vi "Remove_spikes_Single_ch.vi"(0 "LDA data":dbl[][](array[numeric]) format="%.3f", 1 "Sigma cut":i32, 2 "BSA Channels":T1(array[ring]), 3 "LDA numder":enum16{"LDA 1", "LDA 2"}(ring)) -> (5 "Filtered data":dbl[][](array[numeric]) format="%.3f", 6 "No of points removed":i32)   [LabVIEW 2010]
uses:
  Globals/LDA_meas_global_1.vi
  Globals/LDA_meas_global_2.vi
  <vilib>/Analysis/NI_AALBase.lvlib
panel:
  out "No of points outside range":i32
  out "Sigma":dbl[](array[numeric]) format="%.4f"
  out "Points removed":i32[](array[numeric])
  out "output":dbl[][](graph)
  out "input":dbl[][](graph)
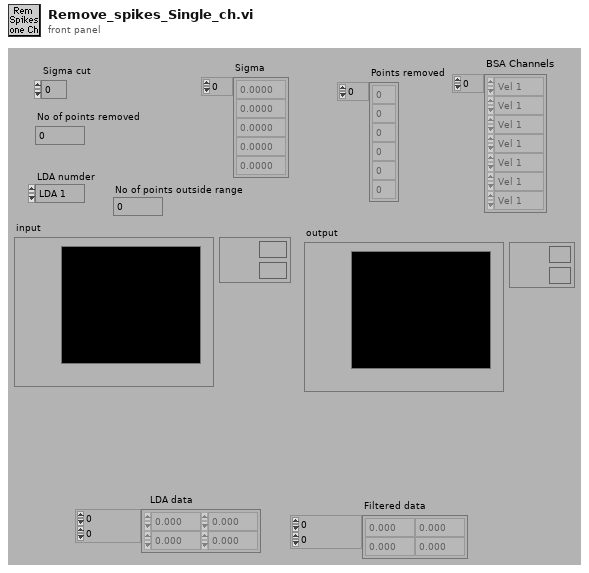
[diagram p1: front panel]
types:
  T1 = enum16{"Vel 1", "Trans 1", "Arr 1", "Vel 2", "Trans 2", "Arr 2", "Index"}[]
  T2 = enum16{"Vel 1", "Trans 1", "Arr 1", "Vel 2", "Trans 2", "Arr 2", "Index"}
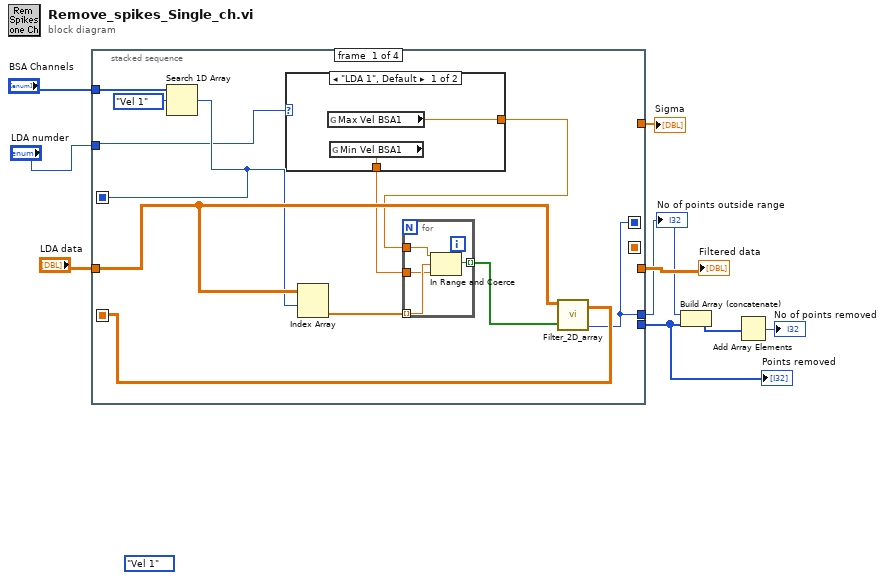
[diagram p0: block diagram]
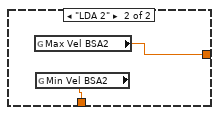
[diagram p2: hidden frame]
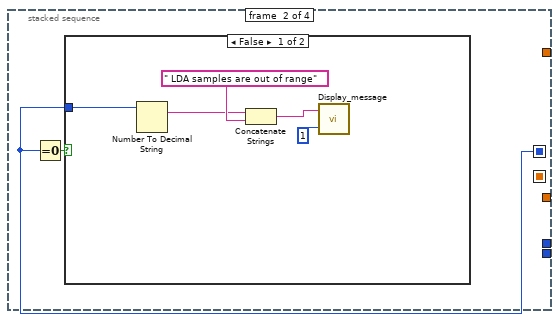
[diagram p3: hidden frame]
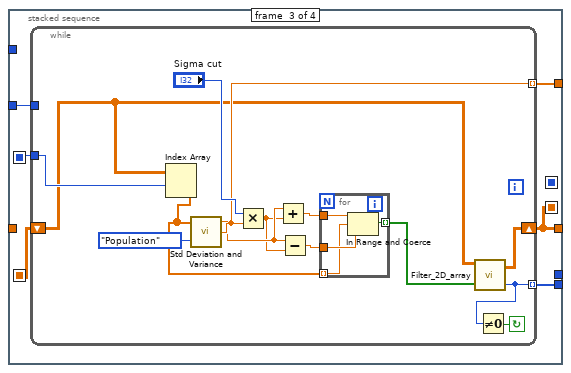
[diagram p5: hidden frame]
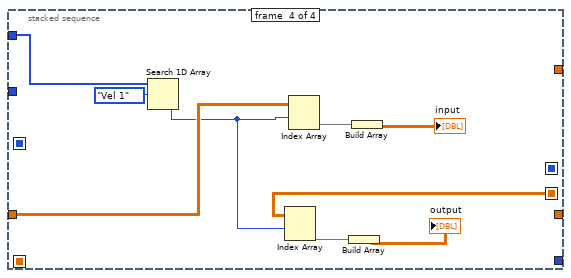
[diagram p6: hidden frame]
diagram:
  (unwired) T2."Vel 1"
  n1 = stacked-sequence {
    seq-local: [w19 _ _ _] -> [_ _ w38 _]
    seq-local: [w18 _ _ _] -> [_ w29 _ _]
    seq-local: [w14 _ _ _] -> [_ _ w37 _]
    seq-local: [_ _ w36 _] -> [_ _ _ w66]
    tunnel: [_ _ w41 _] -> w6
    tunnel: [_ _ w36 _] -> w7
    tunnel: "LDA data" -> [w20 _ _ w67]
    tunnel: [_ _ w40 _] -> w3
    tunnel: "LDA numder" -> [w13 _ w39 _]
    tunnel: [w18 _ _ _] -> w5
    tunnel: "BSA Channels" -> [w17 _ _ w68]
    frame #0 {
      n2 = Search 1D Array(1D array=w17, element=T2."Vel 1") -> (index of element=w14:i32)  [unwired: 1 out]
      n3 = case shown="\"LDA 1\", Default" w13 {
        tunnel: [w22 w24] -> w11
        tunnel: [w21 w23] -> w10
        frame "LDA 1", Default {
          n4 = global read "LDA_meas_global_1.vi" "Max Vel BSA1"() -> (w22:dbl)
          n5 = global read "LDA_meas_global_1.vi" "Min Vel BSA1"() -> (w21:dbl)
        }
        frame "LDA 2" {
          n6 = global read "LDA_meas_global_2.vi" "Max Vel BSA2"() -> (w24:dbl)
          n7 = global read "LDA_meas_global_2.vi" "Min Vel BSA2"() -> (w23:dbl)
        }
      }
      n8 = Index Array(array=w20, index (row)=w14) -> (element=w16:dbl[])  [unwired: 1 in]
      n9 = for {
        tunnel: w16 -> [w28] mode=indexing
        tunnel: [w27] -> w12 mode=indexing
        tunnel: w11 -> [w26]
        tunnel: w10 -> [w25]
        n10 = In Range and Coerce(upper limit=w26, x=w28, lower limit=w25) -> (In Range?=w27:bool)  [unwired: 1 out]
      }
      n11 = call "Filter_2D_array.vi"("All 2D data"=w20, "Accept array"=w12) -> ("Filtered data"=w19:dbl[][], "No of points removed"=w18:i32)  [unwired: 3 out]
    }
    frame #1 {
      n12 = Equal To 0?(x=w29) -> (x = 0?=w30:bool)
      n13 = case shown="False" w30 {
        tunnel: w29 -> [w35 _]
        frame False {
          n14 = Number To Decimal String(number=w35) -> (decimal integer string=w31:string)  [unwired: 1 out]
          n15 = Concatenate Strings(w31, " LDA samples are out of range") -> (w34:string)
          n16 = call "Display_message.vi"("Time to display message"=1, "Message"=w34) -> ()  [unwired: 2 out]
        }
        frame True {
        }
      }
    }
    frame #2 {
      n17 = while {
        tunnel: w37 -> [w50]
        tunnel: [w51] -> w41 mode=indexing
        tunnel: [w53] -> w40 mode=indexing
        tunnel: w39 -> [_]
        shift-left: w38 -> [w49]
        shift-right: [w55] -> w36
        stop <- w54 continue-if-true
        n18 = Index Array(array=w49, index (row)=w50) -> (element=w44:dbl[])  [unwired: 1 in]
        n19 = call <vilib>:"Std Deviation and Variance.vi"("X"=w44, "Weighting (Sample)"=enum16{"Sample", "Population"}."Population") -> ("mean"=w48:dbl, "standard deviation"=w51:dbl)  [unwired: 1 out]
        n20 = Multiply(x="Sigma cut", y=w51) -> (x*y=w45:dbl)
        n21 = Add(x=w48, y=w45) -> (x+y=w46:dbl)
        n22 = Subtract(x=w48, y=w45) -> (x-y=w47:dbl)
        n23 = for {
          tunnel: w46 -> [w59]
          tunnel: w47 -> [w58]
          tunnel: w44 -> [w57] mode=indexing
          tunnel: [w56] -> w43 mode=indexing
          n24 = In Range and Coerce(upper limit=w59, x=w57, lower limit=w58) -> (In Range?=w56:bool)  [unwired: 1 out]
        }
        n25 = call "Filter_2D_array.vi"("All 2D data"=w49, "Accept array"=w43) -> ("Filtered data"=w55:dbl[][], "No of points removed"=w53:i32)  [unwired: 3 out]
        n26 = Not Equal To 0?(x=w53) -> (x != 0?=w54:bool)
      }
    }
    frame #3 {
      n27 = Search 1D Array(1D array=w68, element=T2."Vel 1") -> (index of element=w62:i32)  [unwired: 1 out]
      n28 = Index Array(array=w66, index (row)=w62) -> (element=w60:dbl[])  [unwired: 1 in]
      n29 = Index Array(array=w67, index (row)=w62) -> (element=w61:dbl[])  [unwired: 1 in]
      n30 = Build Array(w60) -> (→"output":dbl[][])
      n31 = Build Array(w61) -> (→"input":dbl[][])
    }
  }
  "Filtered data" <- w7
  "Points removed" <- w3
  "Sigma" <- w6
  "No of points outside range" <- w5
  n32 = Build Array (concatenate)(w5, w3) -> (w4:i32[])
  n33 = Add Array Elements(numeric array=w4) -> (sum=→"No of points removed":i32)
